vi "select drivable paths (behavior).vi"(3 "possible drive vectors":i8[](array[numeric])=[0, 0, 0, 0, 0, 0, 0, 0, 0], 5 "LIDAR Data":T1) -> (1 "driveable drive vectors":i8[](array[numeric]))   [LabVIEW 2009]
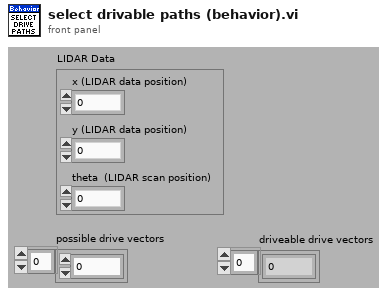
[diagram p1: front panel]
types:
  T1 = cluster{"x (LIDAR data position)":i16, "y (LIDAR data position) ":i16, "theta  (LIDAR scan position)":u8}
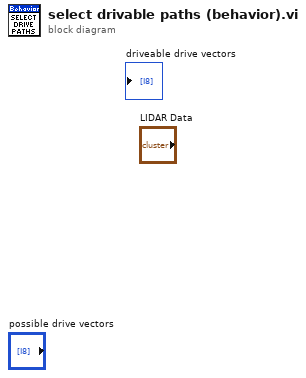
[diagram p0: block diagram]
diagram:
